vi "test json to variant example.vi"(8 "error in (no error)":errorcluster) -> (0 "error out":errorcluster)   [LabVIEW 2019, in "labview_json_tests.lvlib"]
uses:
  labview_json_tests.lvlib
  lib/Element.ctl
  lib/Element Type.ctl
  lib/labview_json.lvlib
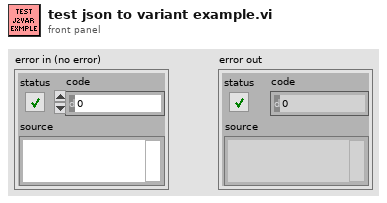
[diagram p1: front panel]
types:
  T1 = typedef "labview_json.lvlib/Element.ctl" = cluster{"Key":string, "Type":T2, "Value":variant, "IsRootPath":bool}
  T2 = typedef "labview_json.lvlib/Element Type.ctl" = enum8{"NULL", "OBJECT", "ARRAY", "BOOL", "INT", "UINT", "FLOAT", "STRING"}
  T3 = cluster{"active":bool, "formed":i32, "homeTown":T1}
  T4 = cluster{"homeTown":string, "formed":i32, "active":bool, "members":cluster{"age":i32, "powers":string[]}[]}
  T5 = cluster{"name":string, "age":i32, "secretIdentity":string, "powers":string[]}
  T6 = cluster{"squadName":string, "homeTown":string, "formed":i32, "secretBase":string, "active":bool, "members":cluster{"name":string, "age":i32, "secretIdentity":string, "powers":string[]}[]}
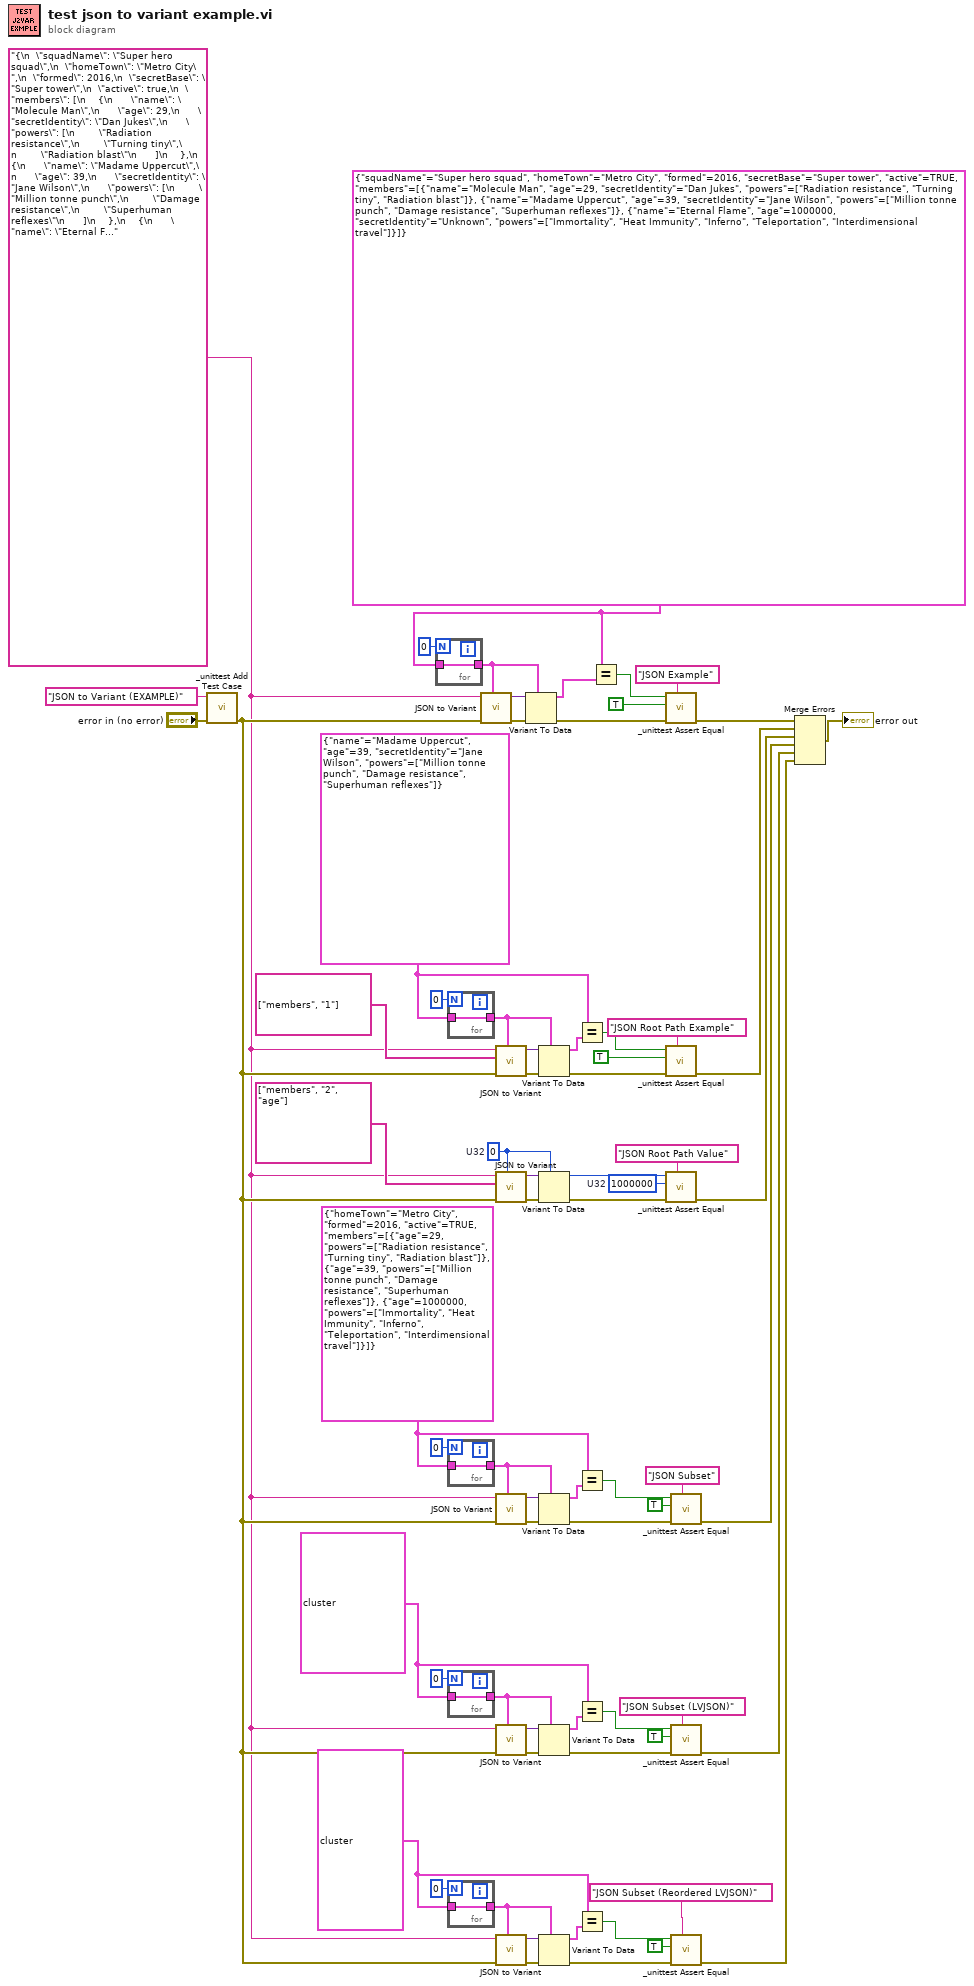
[diagram p0: block diagram]
diagram:
  w13 = T3 {"active"=TRUE, "formed"=2016, "homeTown"={"Key"="homeTown", "Type"=enum."STRING", "Value"=variant(string "Metro City"), "IsRootPath"=FALSE}} ("Root")
  w24 = cluster{"homeTown":string, "members":T1[]} {"homeTown"="Metro City", "members"=[{"Key"="", "Type"=enum."OBJECT", "Value"=variant(cluster{"Key":string, "Type":enum8{"NULL", "OBJECT", "ARRAY", "BOOL", "INT", "UINT", "FLOAT", "STRING"}, "Value":variant, "IsRootPath":bool}[] [{"Key"="name", "Type"=enum."STRING", "Value"=variant(string "Molecule Man"), "IsRootPath"=FALSE}, {"Key"="age", "Type"=enum."UINT", "Value"=variant(u64 29), "IsRootPath"=FALSE}, {"Key"="secretIdentity", "Type"=enum."STRING", "Value"=variant(string "Dan Jukes"), "IsRootPath"=FALSE}, {"Key"="powers", "Type"=enum."ARRAY", "Value"=variant(cluster{"Key":string, "Type":enum8{"NULL", "OBJECT", "ARRAY", "BOOL", "INT", "UINT", "FLOAT", "STRING"}, "Value":variant, "IsRootPath":bool}[] [{"Key"="", "Type"=enum."STRING", "Value"=variant(string "Radiation resistance"), "IsRootPath"=FALSE}, {"Key"="", "Type"=enum."STRING", "Value"=variant(string "Turning tiny"), "IsRootPath"=FALSE}, {"Key"="", "Type"=enum."STRING", "Value"=variant(string "Radiation blast"), "IsRootPath"=FALSE}]), "IsRootPath"=FALSE}]), "IsRootPath"=FALSE}, {"Key"="", "Type"=enum."OBJECT", "Value"=variant(cluster{"Key":string, "Type":enum8{"NULL", "OBJECT", "ARRAY", "BOOL", "INT", "UINT", "FLOAT", "STRING"}, "Value":variant, "IsRootPath":bool}[] [{"Key"="name", "Type"=enum."STRING", "Value"=variant(string "Madame Uppercut"), "IsRootPath"=FALSE}, {"Key"="age", "Type"=enum."UINT", "Value"=variant(u64 39), "IsRootPath"=FALSE}, {"Key"="secretIdentity", "Type"=enum."STRING", "Value"=variant(string "Jane Wilson"), "IsRootPath"=FALSE}, {"Key"="powers", "Type"=enum."ARRAY", "Value"=variant(cluster{"Key":string, "Type":enum8{"NULL", "OBJECT", "ARRAY", "BOOL", "INT", "UINT", "FLOAT", "STRING"}, "Value":variant, "IsRootPath":bool}[] [{"Key"="", "Type"=enum."STRING", "Value"=variant(string "Million tonne punch"), "IsRootPath"=FALSE}, {"Key"="", "Type"=enum."STRING", "Value"=variant(string "Damage resistance"), "IsRootPath"=FALSE}, {"Key"="", "Type"=enum."STRING", "Value"=variant(string "Superhuman reflexes"), "IsRootPath"=FALSE}]), "IsRootPath"=FALSE}]), "IsRootPath"=FALSE}, {"Key"="", "Type"=enum."OBJECT", "Value"=variant(cluster{"Key":string, "Type":enum8{"NULL", "OBJECT", "ARRAY", "BOOL", "INT", "UINT", "FLOAT", "STRING"}, "Value":variant, "IsRootPath":bool}[] [{"Key"="name", "Type"=enum."STRING", "Value"=variant(string "Eternal Flame"), "IsRootPath"=FALSE}, {"Key"="age", "Type"=enum."UINT", "Value"=variant(u64 1000000), "IsRootPath"=FALSE}, {"Key"="secretIdentity", "Type"=enum."STRING", "Value"=variant(string "Unknown"), "IsRootPath"=FALSE}, {"Key"="powers", "Type"=enum."ARRAY", "Value"=variant(cluster{"Key":string, "Type":enum8{"NULL", "OBJECT", "ARRAY", "BOOL", "INT", "UINT", "FLOAT", "STRING"}, "Value":variant, "IsRootPath":bool}[] [{"Key"="", "Type"=enum."STRING", "Value"=variant(string "Immortality"), "IsRootPath"=FALSE}, {"Key"="", "Type"=enum."STRING", "Value"=variant(string "Heat Immunity"), "IsRootPath"=FALSE}, {"Key"="", "Type"=enum."STRING", "Value"=variant(string "Inferno"), "IsRootPath"=FALSE}, {"Key"="", "Type"=enum."STRING", "Value"=variant(string "Teleportation"), "IsRootPath"=FALSE}, {"Key"="", "Type"=enum."STRING", "Value"=variant(string "Interdimensional travel"), "IsRootPath"=FALSE}]), "IsRootPath"=FALSE}]), "IsRootPath"=FALSE}]} ("Root")
  w25 = T4 {"homeTown"="Metro City", "formed"=2016, "active"=TRUE, "members"=[{"age"=29, "powers"=["Radiation resistance", "Turning tiny", "Radiation blast"]}, {"age"=39, "powers"=["Million tonne punch", "Damage resistance", "Superhuman reflexes"]}, {"age"=1000000, "powers"=["Immortality", "Heat Immunity", "Inferno", "Teleportation", "Interdimensional travel"]}]} ("Root")
  w42 = u32 1000000  # U32
  w45 = u32 0  # U32
  w37 = T5 {"name"="Madame Uppercut", "age"=39, "secretIdentity"="Jane Wilson", "powers"=["Million tonne punch", "Damage resistance", "Superhuman reflexes"]} ("member")
  w40 = T6 {"squadName"="Super hero squad", "homeTown"="Metro City", "formed"=2016, "secretBase"="Super tower", "active"=TRUE, "members"=[{"name"="Molecule Man", "age"=29, "secretIdentity"="Dan Jukes", "powers"=["Radiation resistance", "Turning tiny", "Radiation blast"]}, {"name"="Madame Uppercut", "age"=39, "secretIdentity"="Jane Wilson", "powers"=["Million tonne punch", "Damage resistance", "Superhuman reflexes"]}, {"name"="Eternal Flame", "age"=1000000, "secretIdentity"="Unknown", "powers"=["Immortality", "Heat Immunity", "Inferno", "Teleportation", "Interdimensional travel"]}]} ("Root")
  w2 = "{\n  \"squadName\": \"Super hero squad\",\n  \"homeTown\": \"Metro City\",\n  \"formed\": 2016,\n  \"secretBase\": \"Super tower\",\n  \"active\": true,\n  \"members\": [\n    {\n      \"name\": \"Molecule Man\",\n      \"age\": 29,\n      \"secretIdentity\": \"Dan Jukes\",\n      \"powers\": [\n        \"Radiation resistance\",\n        \"Turning tiny\",\n        \"Radiation blast\"\n      ]\n    },\n    {\n      \"name\": \"Madame Uppercut\",\n      \"age\": 39,\n      \"secretIdentity\": \"Jane Wilson\",\n      \"powers\": [\n        \"Million tonne punch\",\n        \"Damage resistance\",\n        \"Superhuman reflexes\"\n      ]\n    },\n    {\n      \"name\": \"Eternal Flame\",\n      \"age\": 1000000,\n      \"secretIdentity\": \"Unknown\",\n      \"powers\": [\n        \"Immortality\",\n        \"Heat Immunity\",\n        \"Inferno\",\n        \"Teleportation\",\n        \"Interdimensional travel\"\n      ]\n    }\n  ]\n}"
  n1 = call "_unittest Add Test Case.vi"("error in (no error)"="error in (no error)", "Test Case"="JSON to Variant (EXAMPLE)") -> ("error out"=w3:errorcluster)  [unwired: 9 in]
  n2 = for {
    N: 0 -> [_]
    tunnel: w40 -> [w71]
    tunnel: [w71] -> w39
  }
  n3 = for {
    N: 0 -> [_]
    tunnel: w37 -> [w72]
    tunnel: [w72] -> w36
  }
  n4 = for {
    N: 0 -> [_]
    tunnel: w25 -> [w73]
    tunnel: [w73] -> w35
  }
  n5 = for {
    N: 0 -> [_]
    tunnel: w24 -> [w74]
    tunnel: [w74] -> w15
  }
  n6 = for {
    N: 0 -> [_]
    tunnel: w13 -> [w75]
    tunnel: [w75] -> w4
  }
  n7 = call "JSON to Variant.vi"("Variant Type"=w39, "error in (no error)"=w3, "JSON"=w2) -> ("error out"=w67:errorcluster, "Variant out"=w65:variant)  [unwired: 7 in]
  n8 = call "JSON to Variant.vi"("Variant Type"=w36, "error in (no error)"=w3, "Root Path ([]=Root)"=string[] ["members", "1"] ("JSON Path (\"\"=Root)"), "JSON"=w2) -> ("error out"=w55:errorcluster, "Variant out"=w57:variant)  [unwired: 6 in]
  n9 = call "JSON to Variant.vi"("Variant Type"=w45, "error in (no error)"=w3, "Root Path ([]=Root)"=string[] ["members", "2", "age"] ("JSON Path (\"\"=Root)"), "JSON"=w2) -> ("error out"=w48:errorcluster, "Variant out"=w46:variant)  [unwired: 6 in]
  n10 = call "JSON to Variant.vi"("Variant Type"=w35, "error in (no error)"=w3, "JSON"=w2) -> ("error out"=w32:errorcluster, "Variant out"=w30:variant)  [unwired: 7 in]
  n11 = call "JSON to Variant.vi"("Variant Type"=w15, "error in (no error)"=w3, "JSON"=w2) -> ("error out"=w18:errorcluster, "Variant out"=w20:variant)  [unwired: 7 in]
  n12 = call "JSON to Variant.vi"("Variant Type"=w4, "error in (no error)"=w3, "JSON"=w2) -> ("error out"=w7:errorcluster, "Variant out"=w9:variant)  [unwired: 7 in]
  n13 = Variant To Data(error in=w67, type=w39, Variant=w65) -> (data=w63:T6, error out=w66:errorcluster)
  n14 = Variant To Data(error in=w55, type=w36, Variant=w57) -> (data=w58:T5, error out=w56:errorcluster)
  n15 = Variant To Data(error in=w48, type=w45, Variant=w46) -> (data=w44:u32, error out=w47:errorcluster)
  n16 = Variant To Data(error in=w32, type=w35, Variant=w30) -> (data=w29:T4, error out=w31:errorcluster)
  n17 = Variant To Data(error in=w18, type=w15, Variant=w20) -> (data=w21:cluster{"homeTown":string, "members":T1[]}, error out=w19:errorcluster)
  n18 = Variant To Data(error in=w7, type=w4, Variant=w9) -> (data=w10:T3, error out=w8:errorcluster)
  n19 = Equal?(x=w37, y=w58) -> (x = y?=w59:bool)
  n20 = Equal?(x=w25, y=w29) -> (x = y?=w28:bool)
  n21 = Equal?(x=w24, y=w21) -> (x = y?=w22:bool)
  n22 = Equal?(x=w13, y=w10) -> (x = y?=w11:bool)
  n23 = Equal?(x=w40, y=w63) -> (x = y?=w62:bool)
  n24 = call "_unittest Assert Equal.vi"("Message"="JSON Example", "error in (no error)"=w66, "Expected Value"=TRUE, "Actual Value"=w62) -> ("error out"=w64:errorcluster)  [unwired: 7 in]
  n25 = call "_unittest Assert Equal.vi"("Message"="JSON Root Path Example", "error in (no error)"=w56, "Expected Value"=TRUE, "Actual Value"=w59) -> ("error out"=w52:errorcluster)  [unwired: 7 in]
  n26 = call "_unittest Assert Equal.vi"("Message"="JSON Root Path Value", "error in (no error)"=w47, "Expected Value"=w42, "Actual Value"=w44) -> ("error out"=w43:errorcluster)  [unwired: 7 in]
  n27 = call "_unittest Assert Equal.vi"("Message"="JSON Subset", "error in (no error)"=w31, "Expected Value"=TRUE, "Actual Value"=w28) -> ("error out"=w26:errorcluster)  [unwired: 7 in]
  n28 = call "_unittest Assert Equal.vi"("Message"="JSON Subset (LVJSON)", "error in (no error)"=w19, "Expected Value"=TRUE, "Actual Value"=w22) -> ("error out"=w14:errorcluster)  [unwired: 7 in]
  n29 = call "_unittest Assert Equal.vi"("Message"="JSON Subset (Reordered LVJSON)", "error in (no error)"=w8, "Expected Value"=TRUE, "Actual Value"=w11) -> ("error out"=w1:errorcluster)  [unwired: 7 in]
  n30 = Merge Errors(w64, w52, w43, w26, w14, w1) -> (→"error out":errorcluster)
